vi "MT_Tran.vi"(8 "Error In":errorcluster caption="错误输入", 9 "位置(mm)":dbl, 10 "偏移量(μm)":dbl, 11 "脉冲个数":dbl) -> (0 "Error Out":errorcluster caption="错误输出", 1 "脉冲位置":dbl, 2 "脉冲个数":dbl, 3 "位置(mm)":dbl)   [LabVIEW 2020]
panel:
  # "MT\n数据\n转换"
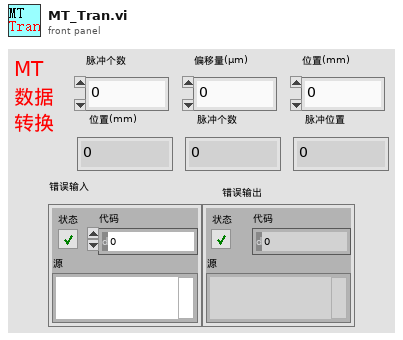
[diagram p1: front panel]
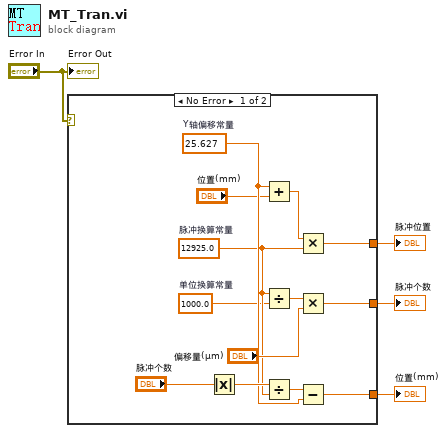
[diagram p0: block diagram]
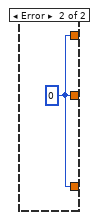
[diagram p2: hidden frame]
diagram:
  n1 = case shown="No Error" "Error In" {
    tunnel: [w12 w18] -> w3
    tunnel: [w5 w18] -> w2
    tunnel: [w6 w18] -> w1
    frame No Error {
      w7 = 1000.0  # 单位换算常量
      w8 = 12925.0  # 脉冲换算常量
      w11 = 25.627  # Y轴偏移常量
      n2 = Absolute Value(x="脉冲个数") -> (abs(x)=w16:dbl)
      n3 = Add(x=w11, y="位置(mm)") -> (x+y=w9:dbl)
      n4 = Divide(x=w8, y=w7) -> (x/y=w14:dbl)
      n5 = Divide(x=w16, y=w8) -> (x/y=w15:dbl)
      n6 = Multiply(x=w9, y=w8) -> (x*y=w6:dbl)
      n7 = Multiply(x=w14, y="偏移量(μm)") -> (x*y=w5:dbl)
      n8 = Subtract(x=w15, y=w11) -> (x-y=w12:dbl)
    }
    frame Error {
      w18 = 0
    }
  }
  "位置(mm)" <- w3
  "脉冲个数" <- w2
  "脉冲位置" <- w1
  "Error Out" <- "Error In"
